vi "Clear Buffer.vi"(8 "error in":errorcluster, 11 "Refnum in":T1) -> (0 "error out":errorcluster, 3 "FPGA VI Reference Out":T1)   [LabVIEW 2015, in "Aircraft OPCCRD.lvclass"]
doc: "Pause the digitization and clear any samples that may be in the buffer. IMPORTANT: Restart the digitizer AFTER this VI is called!!!"
uses:
  Aircraft OPCCRD.lvclass
  tFPGA Ref.ctl
  <vilib>/Utility/error.llb/Error Cluster From Error Code.vi
  <vilib>/rvi/errors/niLvFpgaAdjustHostInterfaceError.vi
  <vilib>/rvi/interface/nirviReadWriteControl/nirviReadWriteControl.xnode
  FPGA Bitfiles/Aircraft OPCRD Server.lvbitx
  <vilib>/rvi/interface/nirviMethod/nirviMethod.xnode
  <vilib>/FPGAPlugInAG/sbRIO-9636/niLvFpga_ReadFifo_sbRIO-9636.vi
  <vilib>/rvi/errors/niLvFpgaMergeErrorWithErrorCode.vi
  NiFpgaLv.dll
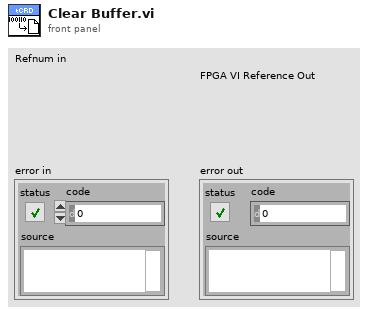
[diagram p1: front panel]
types:
  T1 = typedef "Aircraft OPCCRD.lvclass/tFPGA Ref.ctl" = refnum<k20>
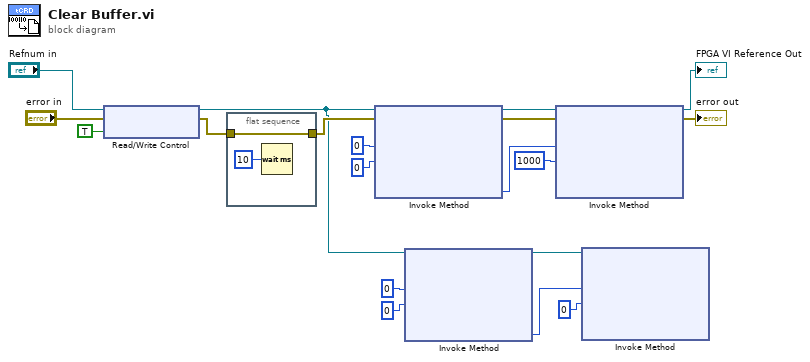
[diagram p0: block diagram]
diagram:
  n1 = xnode "Read/Write Control"("FPGA VI Reference In"="Refnum in", "error in"="error in", "Pause Digitizer"=TRUE) -> ("FPGA VI Reference Out"=w4:T1, "error out"=w8:errorcluster)
  n2 = flat-sequence {
    tunnel: w8 -> [w20]
    tunnel: [w20] -> w7
    frame #0 {
      n3 = Wait (ms)(milliseconds to wait=u32 10) -> ()  [unwired: 1 out]
    }
  }
  n4 = xnode "Invoke Method"("FPGA VI Reference In"=w4, "error in"=w7, "Number of Elements"=u32 0, "Timeout (ms)"=0) -> ("FPGA VI Reference Out"=w13:T1, "error out"=w10:errorcluster, "Elements Remaining"=w12:u32)  [unwired: 1 out]
  n5 = xnode "Invoke Method"("FPGA VI Reference In"=w4, "Number of Elements"=u32 0, "Timeout (ms)"=0) -> ("FPGA VI Reference Out"=w2:T1, "Elements Remaining"=w1:u32)  [unwired: 1 in, 2 out]
  n6 = xnode "Invoke Method"("FPGA VI Reference In"=w13, "error in"=w10, "Number of Elements"=w12, "Timeout (ms)"=1000) -> ("FPGA VI Reference Out"=→"FPGA VI Reference Out":T1, "error out"=→"error out":errorcluster)  [unwired: 2 out]
  n7 = xnode "Invoke Method"("FPGA VI Reference In"=w2, "Number of Elements"=w1, "Timeout (ms)"=0) -> ()  [unwired: 1 in, 4 out]
